vi "Unregister-events.vi"(8 "error in (no error)":errorcluster, 9 "Events":refnum<event-registration>, 11 "Data ref. in":refnum<data-value>) -> (0 "error out":errorcluster, 3 "Data ref.":refnum<data-value>)   [LabVIEW 2013, in "CameraVision.lvlib" / "CV-Main.lvclass"]
uses:
  CV-Main.lvclass
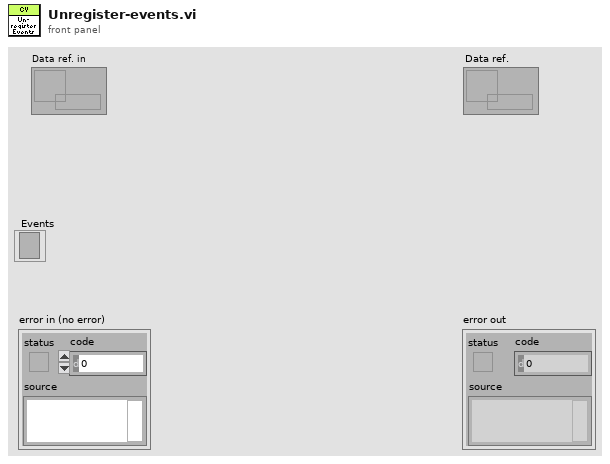
[diagram p1: front panel]
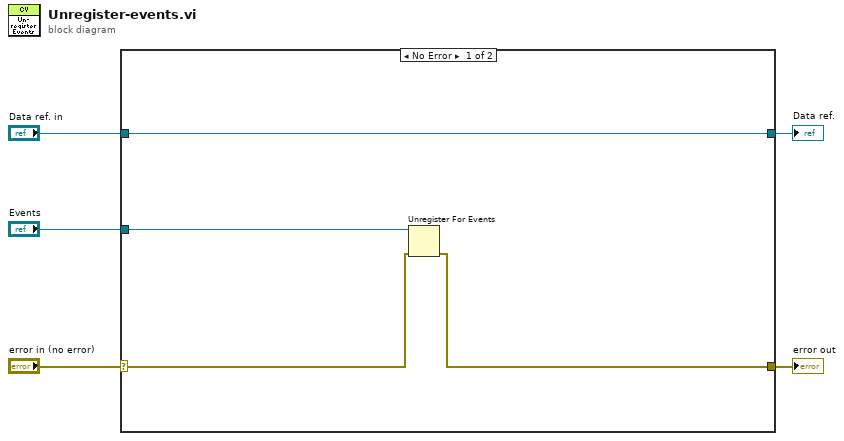
[diagram p0: block diagram]
diagram:
  n1 = case shown="No Error" "error in (no error)" {
    selector: "error in (no error)" -> [w8 w11]
    tunnel: [w7 w11] -> w4
    tunnel: "Data ref. in" -> [w9 w10]
    tunnel: [w9 w10] -> w2
    tunnel: "Events" -> [w6 _]
    frame No Error {
      n2 = Unregister For Events(event registration refnum=w6, error in=w8) -> (error out=w7:errorcluster)
    }
    frame Error {
    }
  }
  "error out" <- w4
  "Data ref." <- w2
